vi "ClientErrorToErrorCluster.vi"(8 "error in (no error)":errorcluster, 10 "ClientError":T1, 11 "response code (200)":T2=200 items=["100"=100, "101"=101, "200"=200, "201"=201, "202"=202, "203"=203, "204"=204, "205"=205, "206"=206, "300"=300, "301"=301, "302"=302, "303"=303, "304"=304, "305"=305, "306"=306, "307"=307, "400"=400, "401"=401, "402"=402, "403"=403, "404"=404, "405"=405, "406"=406, "407"=407, "408"=408, "409"=409, "410"=410, "411"=411, "412"=412, "413"=413, "414"=414, "415"=415, "416"=416, "417"=417, "500"=500, "501"=501, "502"=502, "503"=503, "504"=504, "505"=505]) -> (0 "error out":errorcluster)   [LabVIEW 2020, in "StashRoyale.lvclass"]
uses:
  StashRoyale.lvclass
  ctl_ErrorCodes.ctl
  ctl_ClientError.ctl
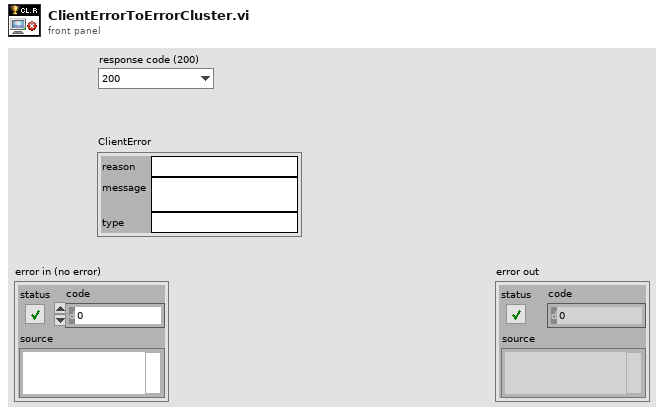
[diagram p1: front panel]
types:
  T1 = typedef "StashRoyale.lvclass/ctl_ClientError.ctl" = cluster{"reason":string, "message":string, "type":string}
  T2 = typedef "StashRoyale.lvclass/ctl_ErrorCodes.ctl" = i32
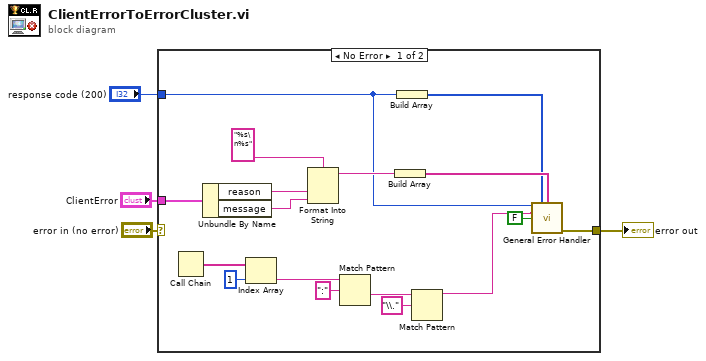
[diagram p0: block diagram]
diagram:
  n1 = case shown="No Error" "error in (no error)" {
    selector: "error in (no error)" -> [_ w22]
    tunnel: "ClientError" -> [w21 _]
    tunnel: [w14 w22] -> w3
    tunnel: "response code (200)" -> [w13 _]
    frame No Error {
      n2 = Call Chain() -> (call chain=w11:string[])
      n3 = Unbundle By Name(w21) -> ("reason"=w20:string, "message"=w19:string)
      n4 = Index Array(array=w11, index=1) -> (element=w9:string)
      n5 = Format Into String(format string="%s\n%s", w20, w19) -> (resulting string=w17:string)  [unwired: 2 in, 1 out]
      n6 = Match Pattern(string=w9, regular expression=":") -> (after substring=w7:string)  [unwired: 1 in, 3 out]
      n7 = Build Array(w17) -> (w16:string[])
      n8 = Build Array(w13) -> (w15:T2[])
      n9 = Match Pattern(string=w7, regular expression="\\.") -> (before substring=w5:string)  [unwired: 1 in, 3 out]
      n10 = call <vilib>:"General Error Handler.vi"("[error code] (0)"=w13, "[user-defined codes]"=w15, "[user-defined descriptions]"=w16, "[error source] (\" \")"=w5, "search ni.com link visible?(T)"=FALSE) -> ("error out"=w14:errorcluster)  [unwired: 6 in, 4 out]
    }
    frame Error {
    }
  }
  "error out" <- w3
